vi "read sync.vi"(8 "error in (no error)":errorcluster, 10 "Number Of Samples":i32, 11 "DeviceRefnum":u64) -> (0 "error out":errorcluster, 1 "Sample Buffer":u8[](array[numeric]), 2 "Samples Read":i32, 3 "DeviceRefnum Out":u64)   [LabVIEW 2015, in "rtlsdr.lvlib"]
doc: "Read a number of samples from the device."
uses:
  rtlsdr.lvlib
  rtlsdr/rtlsdr.dll
panel:
  in  "Sample Buffer In":u8[](array[numeric])
  in  "Samples Read In":i32
  out "function return":i32
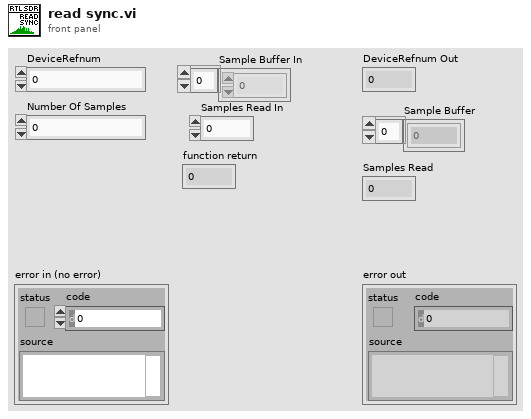
[diagram p1: front panel]
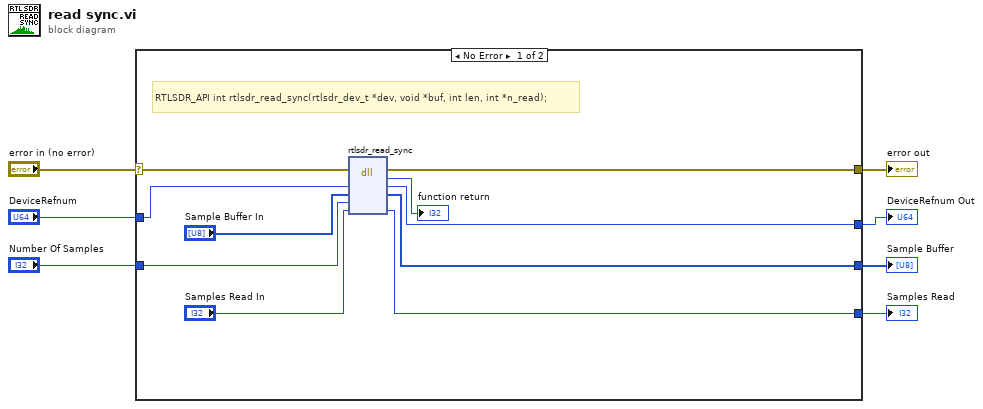
[diagram p0: block diagram]
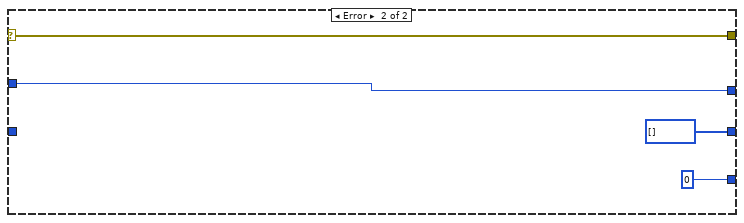
[diagram p2: hidden frame]
diagram:
  n1 = case shown="No Error" "error in (no error)" {
    selector: "error in (no error)" -> [w8 w21]
    tunnel: [w16 u8[] [] ("SampleBuffer")] -> w7
    tunnel: "Number Of Samples" -> [w15 _]
    tunnel: [w13 0 ("SamplesRead")] -> w5
    tunnel: [w12 w21] -> w4
    tunnel: "DeviceRefnum" -> [w11 w19]
    tunnel: [w10 w19] -> w2
    frame No Error {
      # "RTLSDR_API int rtlsdr_read_sync(rtlsdr_dev_t *dev, void *buf, int len, int *n_read);"
      n2 = dll-call lib="C:/Users/TheDoctor/Documents/Projects/Labview Libraries/rtlsdr/rtlsdr.*" fn="rtlsdr_read_sync"(error in=w8, "DeviceRefnum"=w11, "SampleBuffer"="Sample Buffer In", "SamplesToRead"=w15, "SamplesRead"="Samples Read In") -> (error out=w12:errorcluster, "return type"=→"function return":i32, "DeviceRefnum"=w10:u64, "SampleBuffer"=w16:u8[], "SamplesRead"=w13:i32)  [unwired: 3 in, 1 out]
    }
    frame Error {
    }
  }
  "Samples Read" <- w5
  "error out" <- w4
  "DeviceRefnum Out" <- w2
  "Sample Buffer" <- w7
